vi "MsgCfgParser.vi"(1 "search Indexes array":string[](array[string]), 2 "name or relative path":string, 3 "stripped path":path) -> (0 "Msg Cluster Array":cluster{"Names":string[], "Codes":i32[]})   [LabVIEW 2010]
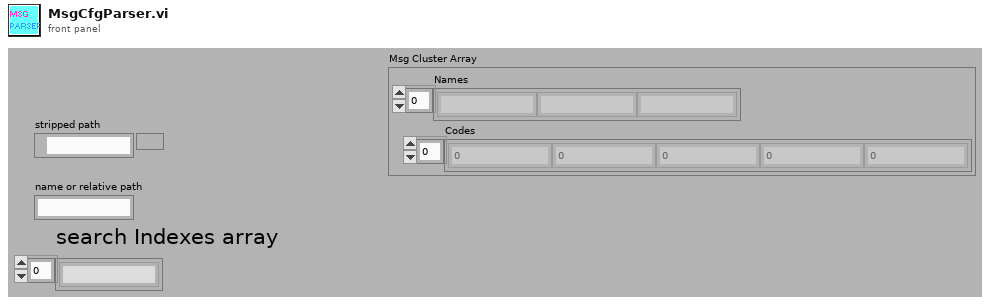
[diagram p1: front panel]
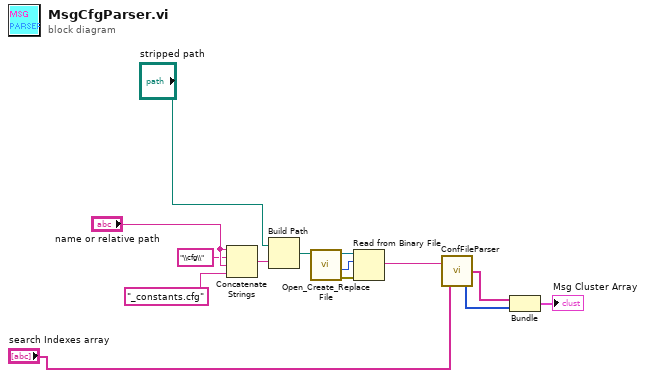
[diagram p0: block diagram]
diagram:
  n1 = Concatenate Strings("name or relative path", "\\cfg\\" ("string"), "name or relative path", "_constants.cfg" ("name or relative path")) -> (w5:string)
  n2 = Build Path(base path="stripped path", name or relative path=w5) -> (appended path=w7:path)
  n3 = call <vilib>:"Open_Create_Replace File.vi"("file path"=w7) -> ("error out"=w8:errorcluster, "file size (bytes)"=w9:i32, "refnum"=w10:refnum<file>)  [unwired: 7 in, 1 out]
  n4 = Read from Binary File(8:w8, 10:w9, 11:w10) -> (2:w13:string)  [unwired: 3 in, 3 out]
  n5 = call "ConfFileParser.vi"("TEXT"=w13, "search Indexes array"="search Indexes array") -> ("Names"=w4:string[], "Codes"=w3:i32[])  [unwired: 1 out]
  n6 = Bundle("Names"=w4, "Codes"=w3) -> (→"Msg Cluster Array":cluster{"Names":string[], "Codes":i32[]})  [unwired: 1 in]
